vi "index.vi"() -> (1 "XY graph visual":cluster{dbl[], dbl[]}(graph))   [LabVIEW 2026]
uses:
  <userlib>/Status.ctl
  <vilib>/Instr/_visa.llb/VISA Flush IO Buffer Mask.ctl
  <vilib>/Instr/_visa.llb/VISA Configure Serial Port (Instr).vi
  <vilib>/Analysis/3filter.llb/Butterworth Filter (DBL).vi
  <vilib>/measure/maspectr.llb/FFT Spectrum (Mag-Phase) for N Chan.vi
  <vilib>/measure/NI_MAPro.lvlib
  <vilib>/Analysis/NI_AALBase.lvlib
panel:
  in  "Okno osy X":dbl(knob) scale=5.0..30.0 scale format="%#_4g"
  in  "DO 2":bool
  in  "DO 1":bool
  in  "Cluster 2":T1={"Zařízení"="", "Cesta k uloženému souboru"=path "", "Vzorkovací frekvence"=enum."1000", "Record Button"=FALSE, "Stop Button"=FALSE, "A1 signál"=enum."EMG", "A2 signál"=enum."EMG", "A3 signál"=enum."EMG", "A4 signál"=enum."EMG", "A5 signál"=enum."EMG", "A6 signál"=enum."EMG", "Pin s připojeným signálem"=enum."A1"}
  out "read buffer":string
  out "CRC Error":bool
  out "Spectrum":cluster{"f0":dbl, "df":dbl, "magnitude":dbl[]}[](graph)
  in  "EditCluster":T2={"Horní mezní frekvence"=0.45000000000000007, "Dolní mezní frekvence"=0.0, "filter type"=enum."Lowpass", "applyFilter"=FALSE, "removeFilter"=FALSE, "undoFIlter"=FALSE} {"Horní mezní frekvence" format="%0.2f"}
  out "Waveform Graph Edit":waveform(dbl)[](graph)
  out "Zobrazeni typu signalu":cluster{string, string}
  in  "Exit Button":bool
  in  "MereniAZpracovaniSwitch":bool
  in  "DO 4":bool
  in  "DO 3":bool
  out "tdms file":refnum<k34>
  out "Ylabel and Plot name":cluster{string, string}
  out "Sample Rate Numeric":i32
  out "Consumer":i32
  out "producer":i32
  in  "error in (no error)":errorcluster
  out "Sync Stop":bool=TRUE
  # "Aplikace pro měření a zpracování dat na platformě PLUX BITalino"
  # "Hz"
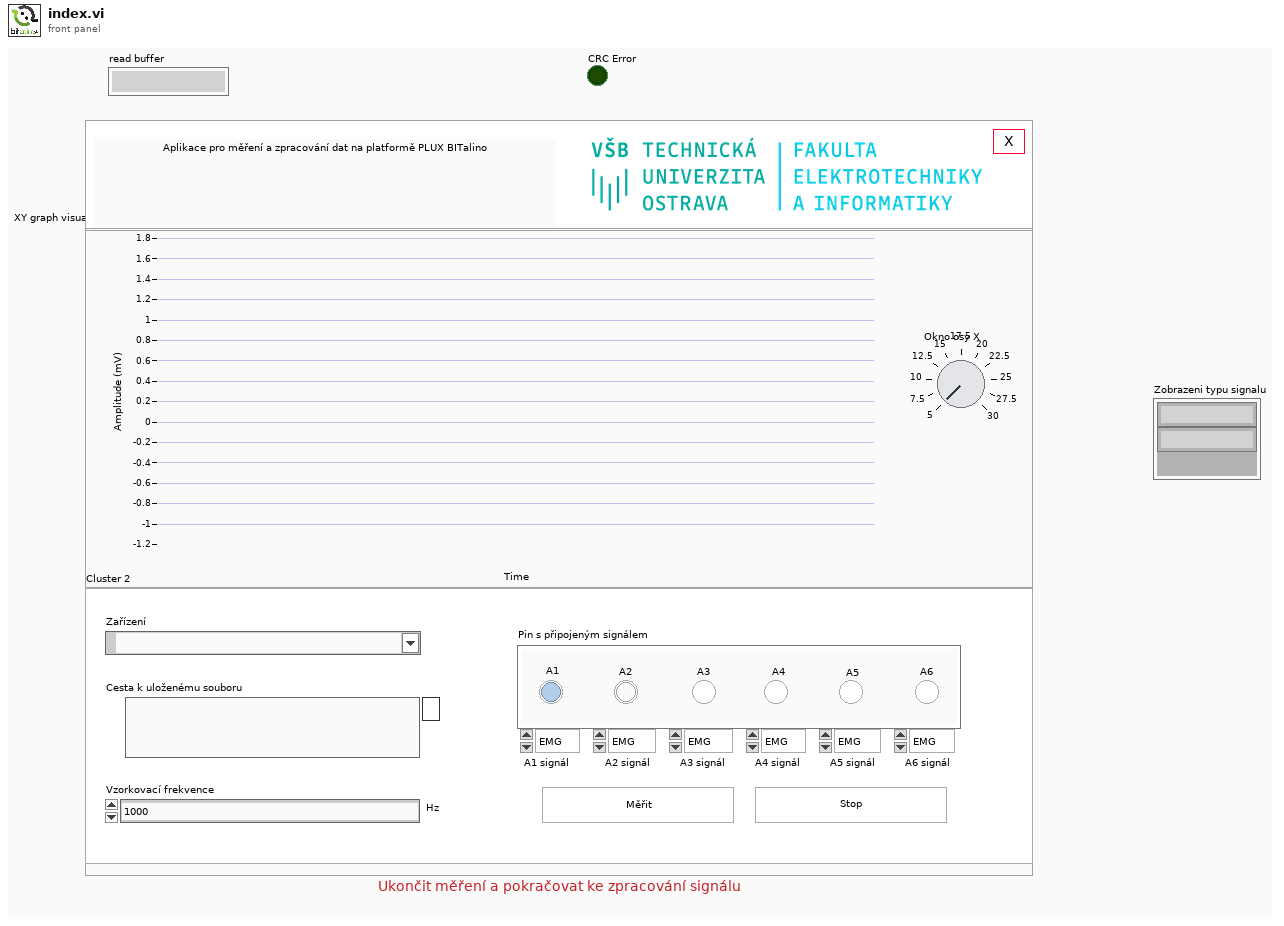
[diagram p1: front panel]
types:
  T1 = cluster{"Zařízení":refnum<visa-resource-name>, "Cesta k uloženému souboru":path, "Vzorkovací frekvence":enum16{"1", "10", "100", "1000"}, "Record Button":bool, "Stop Button":bool, "A1 signál":enum16{"EMG", "ECG", "EEG", "EDA", "ACC"}, "A2 signál":enum16{"EMG", "ECG", "EEG", "EDA", "ACC"}, "A3 signál":enum16{"EMG", "ECG", "EEG", "EDA", "ACC"}, "A4 signál":enum16{"EMG", "ECG", "EEG", "EDA", "ACC"}, "A5 signál":enum16{"EMG", "ECG", "EEG", "EDA", "ACC"}, "A6 signál":enum16{"EMG", "ECG", "EEG", "EDA", "ACC"}, "Pin s připojeným signálem":enum32{"A1", "A2", "A3", "A4", "A5", "A6"}}
  T2 = cluster{"Horní mezní frekvence":dbl, "Dolní mezní frekvence":dbl, "filter type":enum32{"Lowpass", "Highpass", "Bandpass", "Bandstop"}, "applyFilter":bool, "removeFilter":bool, "undoFIlter":bool}
  T3 = enum8{"Enabled", "Disabled", "Disabled and Grayed Out"}
  T4 = enum16{"open", "open or create", "create or replace", "create", "open (read-only)"}
  T5 = typedef "Status.ctl" = enum16{"Initialize", "Edit", "Standby", "Recording", "Exit"}
  T6 = typedef "VISA Flush IO Buffer Mask.ctl" = u16
  T7 = enum32{"Lowpass", "Highpass", "Bandpass", "Bandstop"}
  T8 = cluster{"A1 signál":enum16{"EMG", "ECG", "EEG", "EDA", "ACC"}, "A2 signál":enum16{"EMG", "ECG", "EEG", "EDA", "ACC"}, "A3 signál":enum16{"EMG", "ECG", "EEG", "EDA", "ACC"}, "A4 signál":enum16{"EMG", "ECG", "EEG", "EDA", "ACC"}, "A5 signál":enum16{"EMG", "ECG", "EEG", "EDA", "ACC"}, "A6 signál":enum16{"EMG", "ECG", "EEG", "EDA", "ACC"}}
  T9 = cluster{"Result":dbl, "Result":dbl, "Result":dbl, "Result":dbl, "Result":dbl, "Result":dbl}
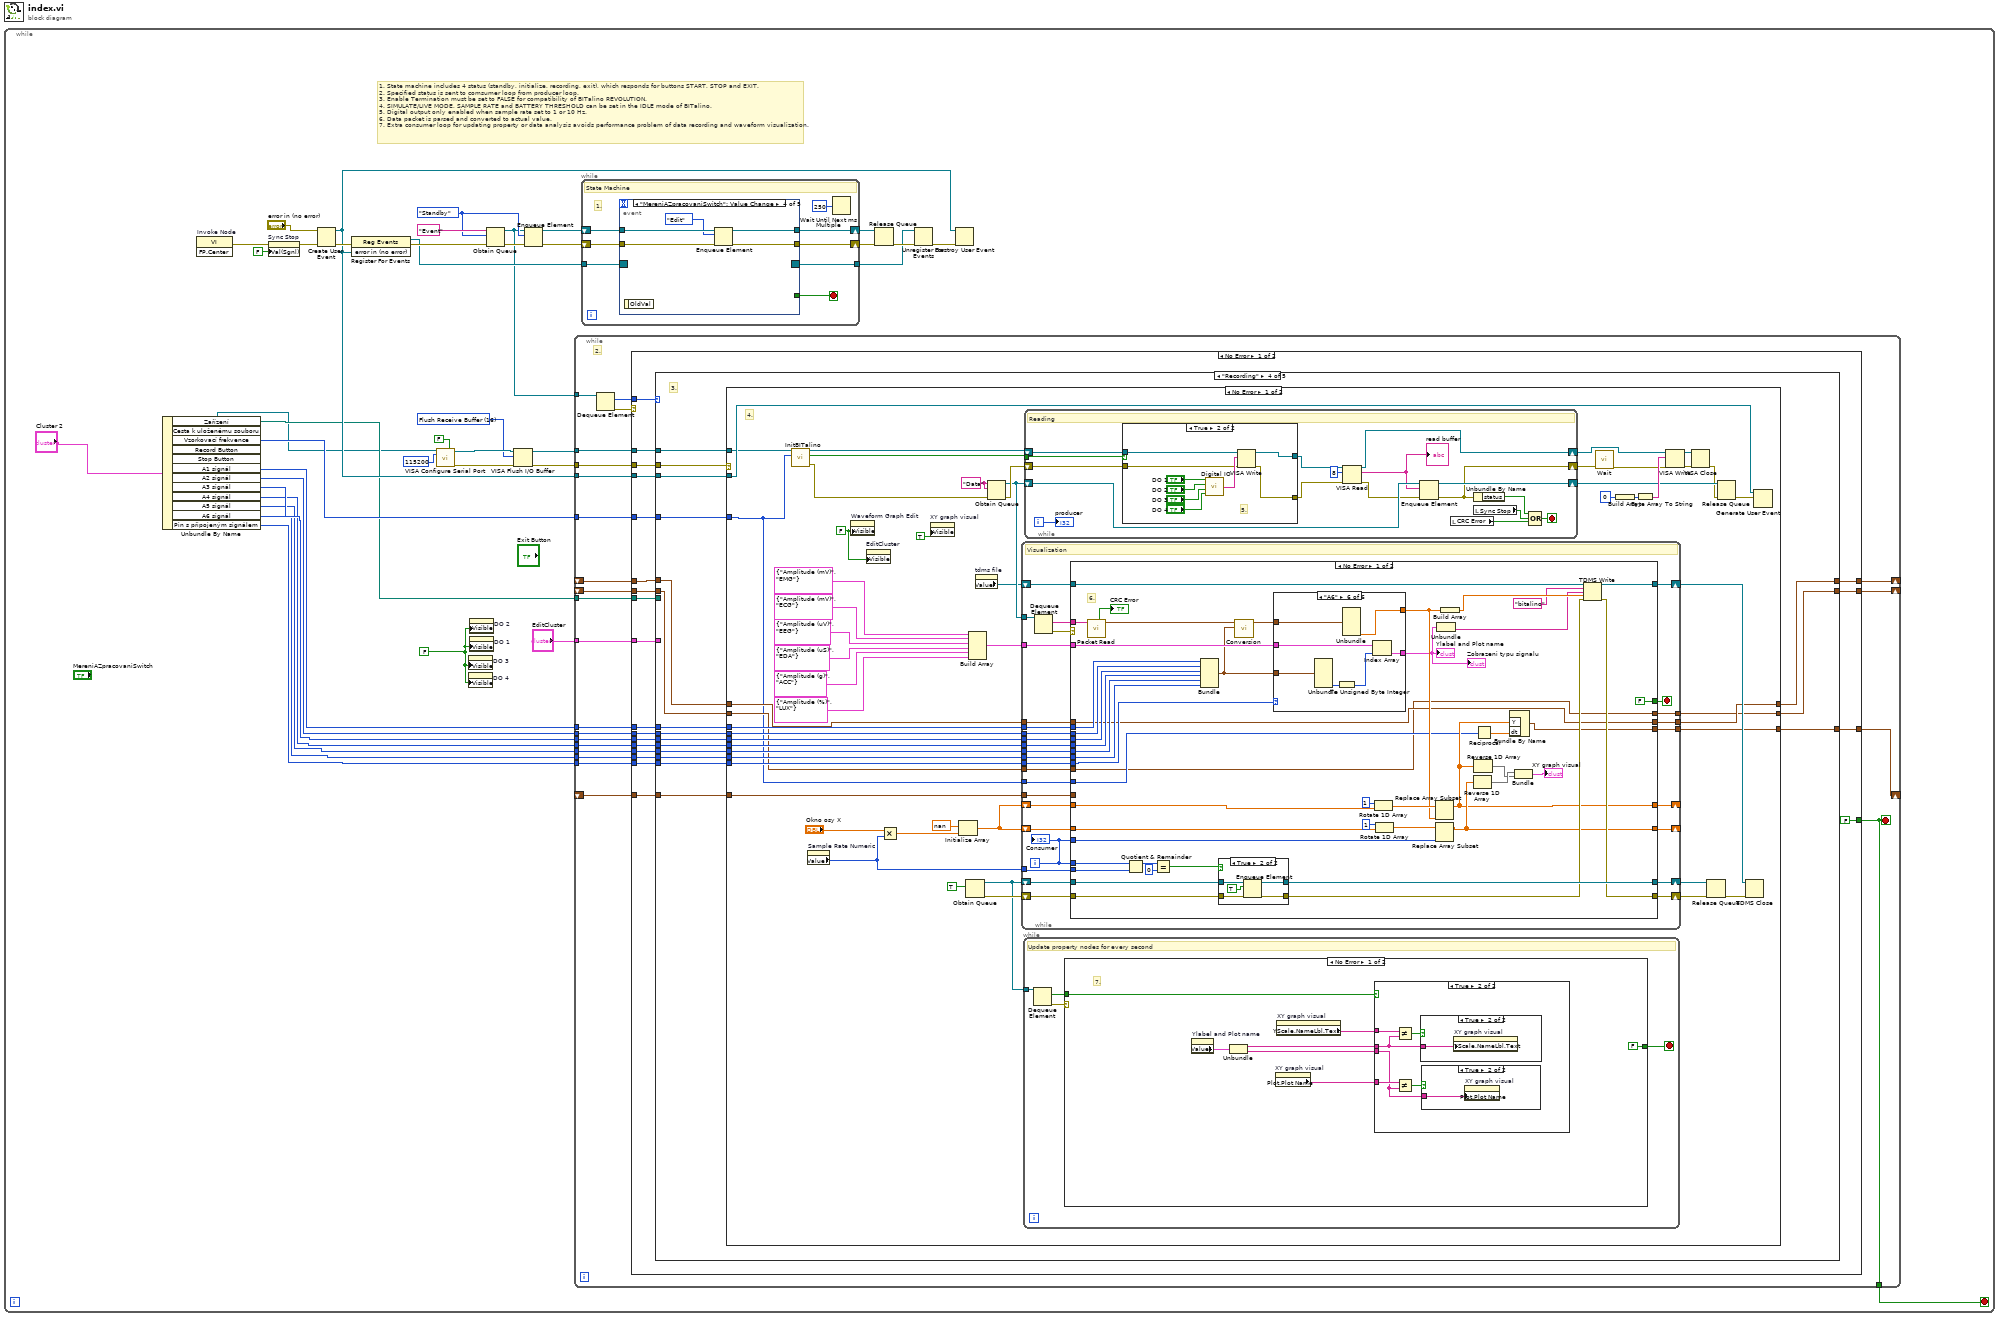
[diagram p0: block diagram]
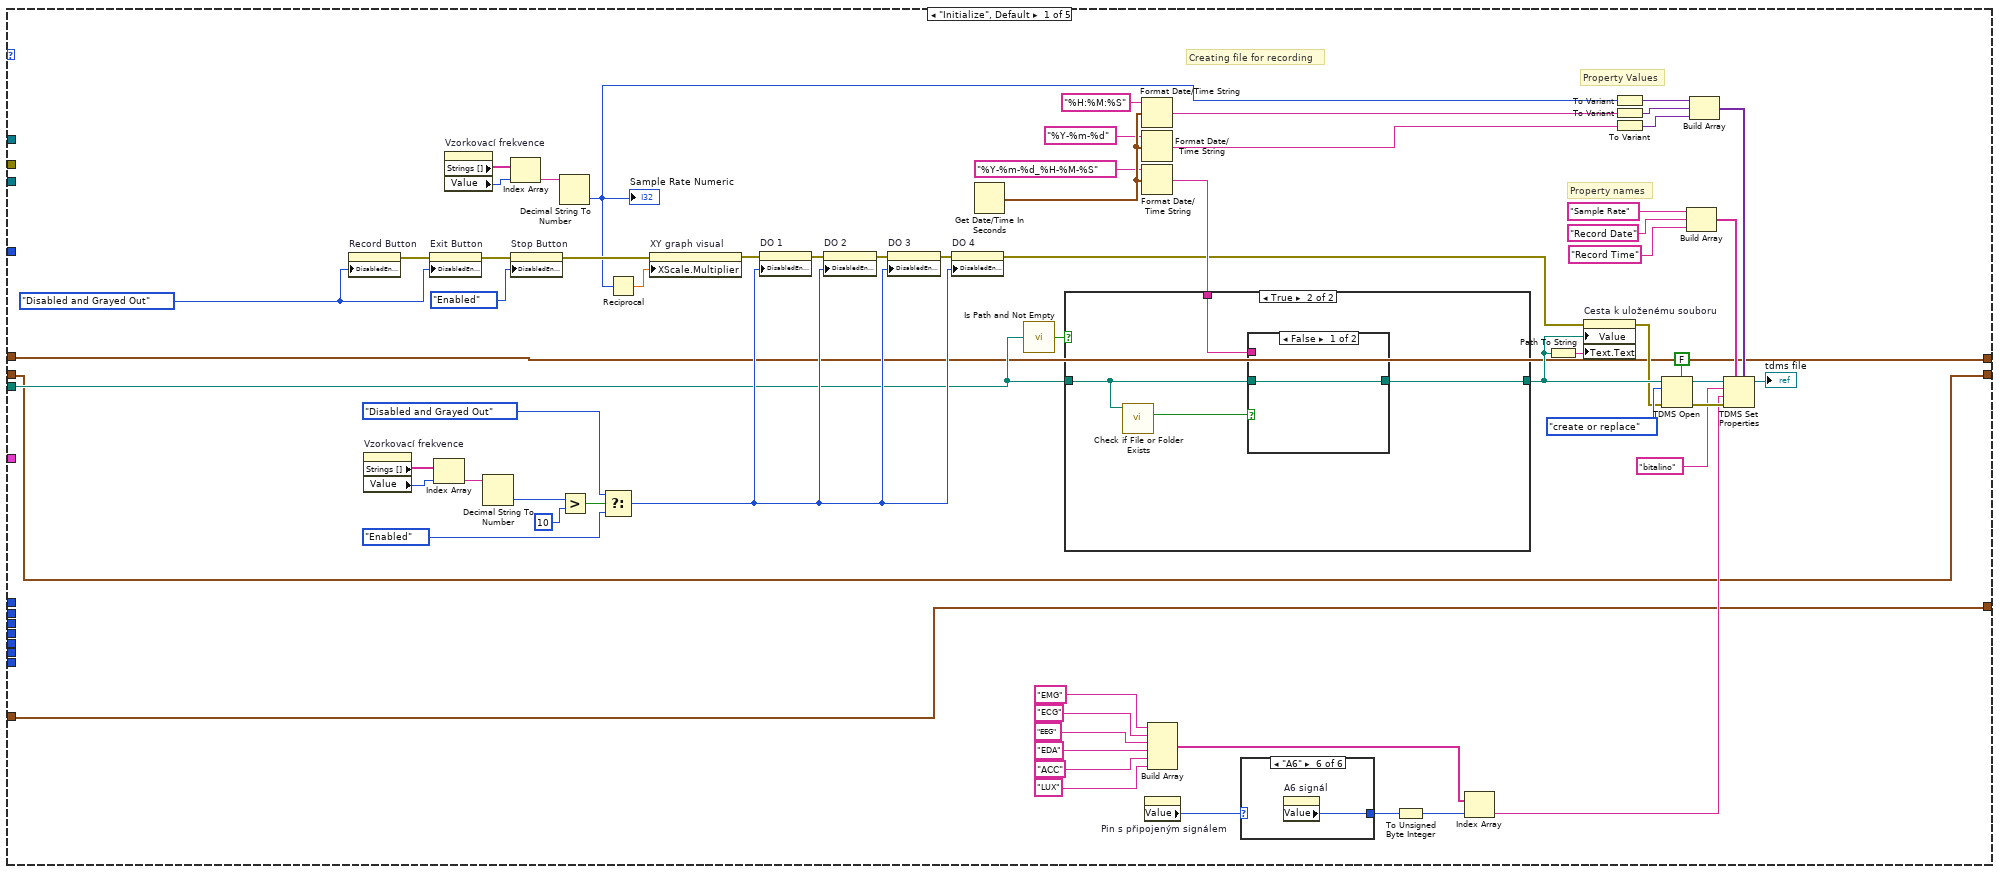
[diagram p2: hidden frame]
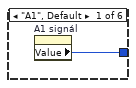
[diagram p3: hidden frame]
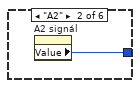
[diagram p4: hidden frame]
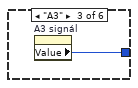
[diagram p5: hidden frame]
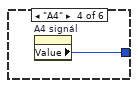
[diagram p6: hidden frame]
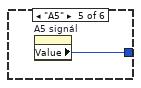
[diagram p7: hidden frame]
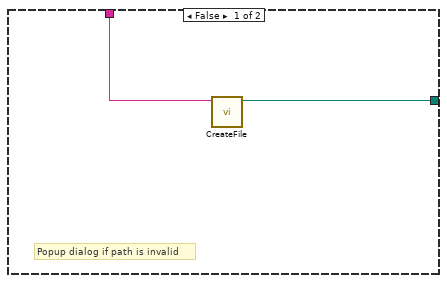
[diagram p8: hidden frame]
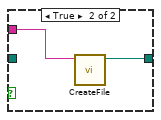
[diagram p9: hidden frame]
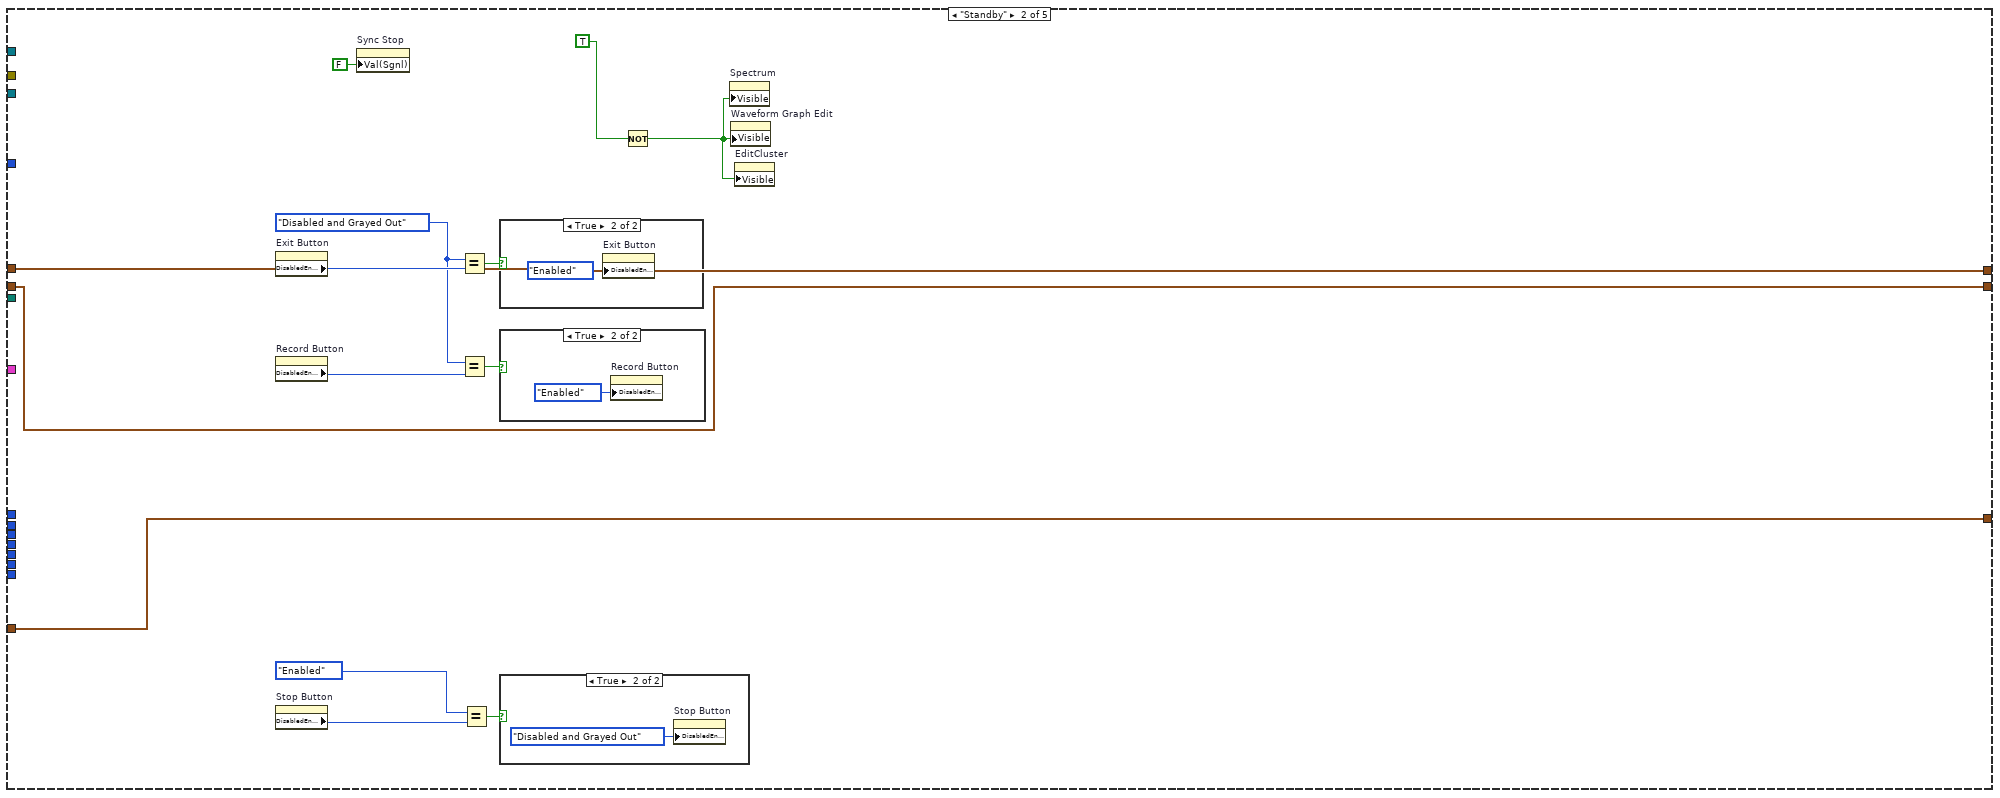
[diagram p10: hidden frame]
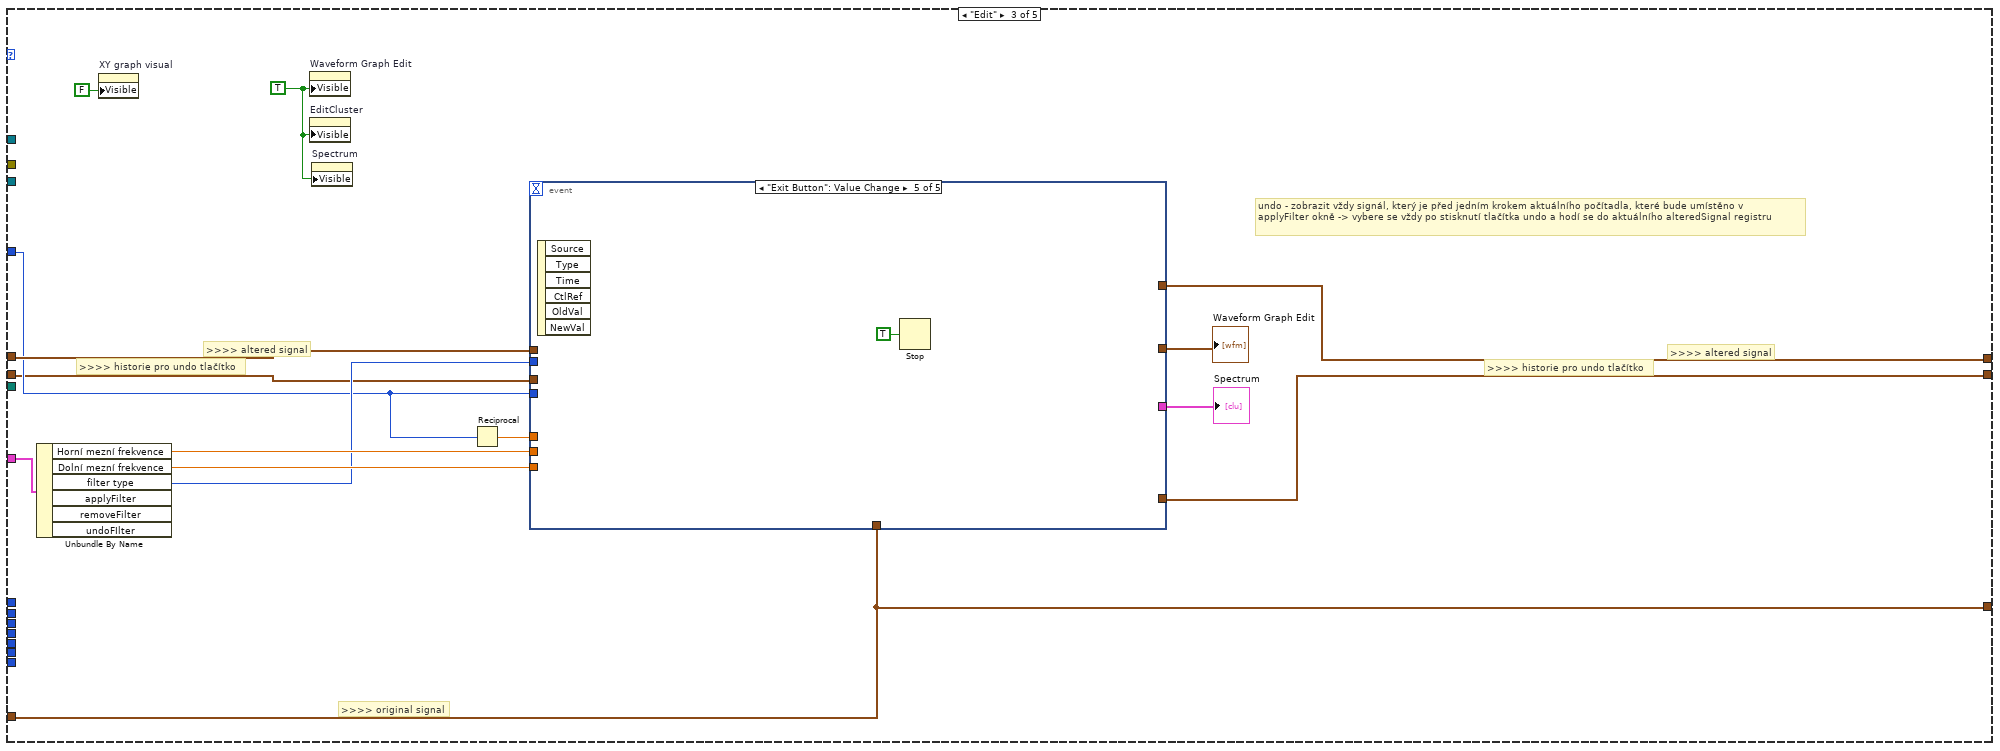
[diagram p14: hidden frame]
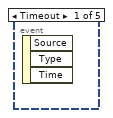
[diagram p15: hidden frame]
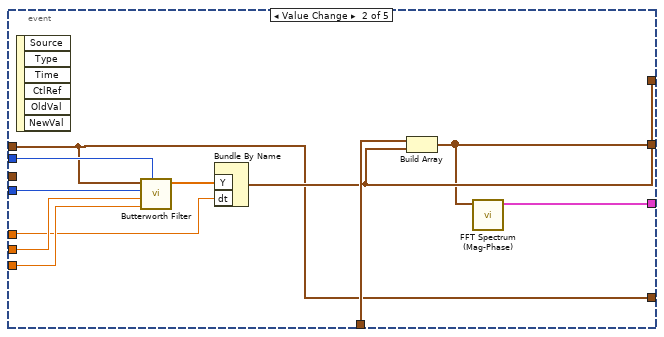
[diagram p16: hidden frame]
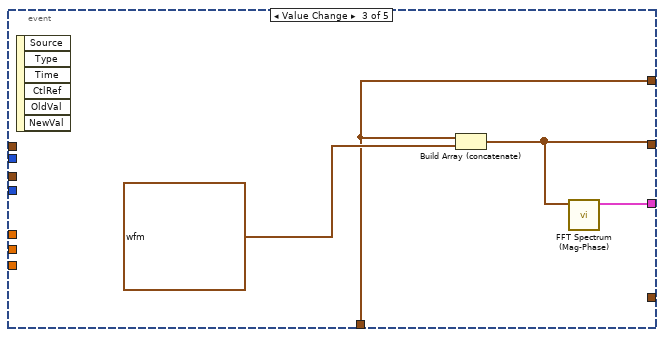
[diagram p17: hidden frame]
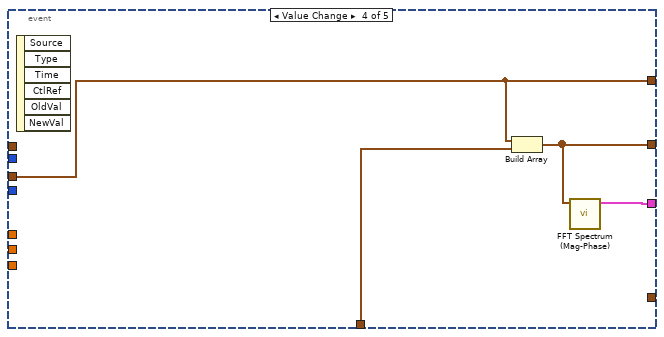
[diagram p18: hidden frame]
diagram:
  n1 = while {
    stop <- w12 stop-if-true
    w1 = FALSE
    w3 = T6 16 items=["Flush Receive Buffer"=16, "Write Transmit Buffer to Device"=32, "Flush Receive Buffer (No I/O)"=64, "Flush Transmit Buffer"=128] ("Mask")
    w39 = Status."Standby" ("Enum")
    # "1. State machine includes 4 status (standby, initialize, recording, exit), which responds for buttons START, STOP and EXIT.\n2. Specified status is sent to comsumer loop from producer loop.\n3. Enable Termination must be set to FALSE for compatibility of BITalino REVOLUTION.\n4. SIMULATE/LIVE MODE, SAMPLE RATE and BATTERY THRESHOLD can be set in the IDLE mode of BITalino.\n5. Digital output only enabled when sample rate set to 1 or 10 Hz.\n6. Data packet is parsed and converted to actual value.\n7. Extra consumer loop for updating property or data analysis avoids performance problem of data recording and waveform visualization."
    n2 = Unbundle By Name("Cluster 2") -> ("Zařízení"=w10:refnum<visa-resource-name>, "Cesta k uloženému souboru"=w13:path, "Vzorkovací frekvence"=w21:enum16{"1", "10", "100", "1000"}, "A1 signál"=w20:enum16{"EMG", "ECG", "EEG", "EDA", "ACC"}, "A2 signál"=w19:enum16{"EMG", "ECG", "EEG", "EDA", "ACC"}, "A3 signál"=w18:enum16{"EMG", "ECG", "EEG", "EDA", "ACC"}, "A4 signál"=w17:enum16{"EMG", "ECG", "EEG", "EDA", "ACC"}, "A5 signál"=w16:enum16{"EMG", "ECG", "EEG", "EDA", "ACC"}, "A6 signál"=w15:enum16{"EMG", "ECG", "EEG", "EDA", "ACC"}, "Pin s připojeným signálem"=w14:enum32{"A1", "A2", "A3", "A4", "A5", "A6"})  [unwired: 2 out]
    n3 = invoke on="Invoke Node" class="VI" method="FP.Center"() -> (error out=w23:errorcluster)  [unwired: 3 in, 2 out]
    n4 = property on="Sync Stop" class="Bool (strict)"(error in=w23, "Val(Sgnl)"=FALSE ("Value (Signaling)")) -> (error out=w32:errorcluster)  [unwired: 1 in, 1 out]
    n5 = Create User Event(user event datatype="error in (no error)", error in=w32) -> (user event=w24:refnum<user-event>, error out=w31:errorcluster)
    n6 = register-events(error in=w31, w24) -> (reference out=w29:refnum<event-registration>, error out=w30:errorcluster)  [unwired: 1 in]
    n7 = call-poly "VISA Configure Serial Port"("VISA resource name"=w10, "Enable Termination\nChar (T)"=FALSE ("Enable Termination\nChar (T)"), "baud rate (9600)"=u32 115200) -> ("VISA resource name out"=w7:refnum<visa-resource-name>, "error out"=w6:errorcluster)  [unwired: 11 in]
    n8 = property on="DO 3" class="Bool (strict)"("Visible"=w1) -> ()  [unwired: 2 in, 2 out]
    n9 = property on="DO 4" class="Bool (strict)"("Visible"=w1) -> ()  [unwired: 2 in, 2 out]
    n10 = property on="DO 2" class="Bool (strict)"("Visible"=w1) -> ()  [unwired: 2 in, 2 out]
    n11 = property on="DO 1" class="Bool (strict)"("Visible"=w1) -> ()  [unwired: 2 in, 2 out]
    n12 = Obtain Queue(name (unnamed)="Event", element data type=w39, error in (no error)=w30) -> (queue out=w22:refnum<queue>, error out=w35:errorcluster)  [unwired: 2 in, 1 out]
    n13 = VISA Flush I/O Buffer(VISA resource name=w7, mask (16)=w3, error in (no error)=w6) -> (VISA resource name out=w5:refnum<visa-resource-name>, error out=w4:errorcluster)
    n14 = Enqueue Element(queue=w22, element=w39, error in (no error)=w35) -> (queue out=w33:refnum<queue>, error out=w34:errorcluster)  [unwired: 1 in, 1 out]
    n15 = while {
      tunnel: w22 -> [w63]
      tunnel: w24 -> [w43]
      tunnel: w21 -> [w60]
      tunnel: [w59] -> w12
      tunnel: w20 -> [w58]
      tunnel: w19 -> [w57]
      tunnel: w18 -> [w56]
      tunnel: w17 -> [w55]
      tunnel: w16 -> [w54]
      tunnel: w15 -> [w53]
      tunnel: w14 -> [w52]
      tunnel: w13 -> [w51]
      shift-right: [w50] -> _
      shift-left: _ -> [w49]
      tunnel: "EditCluster" -> [w48]
      shift-right: [w47] -> _
      shift-left: _ -> [w46]
      shift-right: [w45] -> _
      shift-left: _ -> [w44]
      tunnel: w4 -> [w42]
      tunnel: w5 -> [w41]
      stop <- w59 stop-if-true
      # "2."
      n16 = Dequeue Element(queue=w63) -> (element=w62:T5, error out=w61:errorcluster)  [unwired: 2 in, 2 out]
      n17 = case shown="No Error" w61 {
        tunnel: w62 -> [w82 _]
        tunnel: [FALSE TRUE] -> w59
        tunnel: w60 -> [w83 _]
        tunnel: w58 -> [w81 _]
        tunnel: w57 -> [w80 _]
        tunnel: w56 -> [w79 _]
        tunnel: w55 -> [w78 _]
        tunnel: w54 -> [w77 _]
        tunnel: w53 -> [w76 _]
        tunnel: w52 -> [w75 _]
        tunnel: w51 -> [w74 _]
        tunnel: [w73 w485] -> w50
        tunnel: w49 -> [w72 w485]
        tunnel: w48 -> [w71 _]
        tunnel: [w70 w484] -> w47
        tunnel: w46 -> [w69 w484]
        tunnel: [w68 w483] -> w45
        tunnel: w44 -> [w67 w483]
        tunnel: w43 -> [w66 _]
        tunnel: w42 -> [w65 _]
        tunnel: w41 -> [w64 _]
        frame No Error {
          n18 = case shown="\"Recording\"" w82 {
            tunnel: w83 -> [_ _ w187 w232 _]
            tunnel: w81 -> [_ _ _ w231 _]
            tunnel: w80 -> [_ _ _ w230 _]
            tunnel: w79 -> [_ _ _ w229 _]
            tunnel: w78 -> [_ _ _ w228 _]
            tunnel: w77 -> [_ _ _ w227 _]
            tunnel: w76 -> [_ _ _ w226 _]
            tunnel: w75 -> [_ _ _ w225 _]
            tunnel: w74 -> [w88 _ _ _ _]
            tunnel: [w87 w168 w184 w224 w480] -> w73
            tunnel: w72 -> [w87 w168 w184 w223 w480]
            tunnel: w71 -> [_ _ w194 _ _]
            tunnel: [w86 w167 w183 w222 w479] -> w70
            tunnel: w69 -> [w86 w167 w192 w221 w479]
            tunnel: [w85 w165 w182 w220 w478] -> w68
            tunnel: w67 -> [w85 w165 w181 w219 w478]
            tunnel: w66 -> [_ _ _ w218 _]
            tunnel: w65 -> [_ _ _ w217 _]
            tunnel: w64 -> [_ _ _ w216 _]
            frame "Initialize", Default {
              w116 = T3."Disabled and Grayed Out" ("Disabled")
              # "Creating file for recording"
              # "Property Values"
              # "Property names"
              n19 = property on="Record Button" class="Bool"("DisabledEnum"=w116) -> (error out=w148:errorcluster)  [unwired: 2 in, 1 out]
              n20 = property on="Vzorkovací frekvence" class="Enum (strict)"() -> ("Strings []"=w106:string[], "Value"=w105:enum16{"1", "10", "100", "1000"})  [unwired: 2 in, 2 out]
              n21 = property on="Exit Button" class="Bool"(error in=w148, "DisabledEnum"=w116) -> (error out=w146:errorcluster)  [unwired: 1 in, 1 out]
              n22 = Index Array "Index Array"(array=w106, index=w105) -> (element=w104:string)
              n23 = property on="Vzorkovací frekvence" class="Enum (strict)"() -> ("Strings []"=w145:string[], "Value"=w144:enum16{"1", "10", "100", "1000"})  [unwired: 2 in, 2 out]
              n24 = Decimal String To Number(string=w104) -> (number=w103:i32)  [unwired: 2 in, 1 out]
              n25 = Index Array(array=w145, index=w144) -> (element=w143:string)
              n26 = property on="Stop Button" class="Bool"(error in=w146, "DisabledEnum"=T3."Enabled" ("Disabled")) -> (error out=w142:errorcluster)  [unwired: 1 in, 1 out]
              n27 = Decimal String To Number(string=w143) -> (number=w115:i32)  [unwired: 2 in, 1 out]
              "Sample Rate Numeric" <- w115
              n28 = Greater?(x=w103, y=10) -> (0:w111:bool)
              n29 = Select(t=T3."Disabled and Grayed Out" ("Disabled"), s=w111, f=T3."Enabled" ("Disabled")) -> (s? t:f=w114:T3)
              n30 = Reciprocal(x=w115) -> (1/x=w141:dbl)
              n31 = property on="XY graph visual" class="XYGraph (strict)"(error in=w142, "XScale.Multiplier"=w141) -> (error out=w102:errorcluster)  [unwired: 1 in, 1 out]
              n32 = property on="DO 1" class="Bool (strict)"(error in=w102, "DisabledEnum"=w114) -> (error out=w109:errorcluster)  [unwired: 1 in, 1 out]
              n33 = property on="DO 2" class="Bool (strict)"(error in=w109, "DisabledEnum"=w114) -> (error out=w108:errorcluster)  [unwired: 1 in, 1 out]
              n34 = property on="DO 3" class="Bool (strict)"(error in=w108, "DisabledEnum"=w114) -> (error out=w107:errorcluster)  [unwired: 1 in, 1 out]
              n35 = property on="DO 4" class="Bool (strict)"(error in=w107, "DisabledEnum"=w114) -> (error out=w101:errorcluster)  [unwired: 1 in, 1 out]
              n36 = Get Date/Time In Seconds() -> (seconds since 1Jan1904=w131:timestamp)
              n37 = call <vilib>:"Is Path and Not Empty.vi"("path"=w88) -> ("Is Path and Not Empty?"=w123:bool)  [unwired: 4 in]
              n38 = Format Date/Time String(time format string (%c)="%H:%M:%S", seconds (now)=w131) -> (date/time string=w136:string)  [unwired: 1 in]
              n39 = Format Date/Time String(time format string (%c)="%Y-%m-%d", seconds (now)=w131) -> (date/time string=w137:string)  [unwired: 1 in]
              n40 = Format Date/Time String(time format string (%c)="%Y-%m-%d_%H-%M-%S", seconds (now)=w131) -> (date/time string=w127:string)  [unwired: 1 in]
              n41 = case shown="True" w123 {
                tunnel: [w155 w158] -> w120
                tunnel: w88 -> [_ w157]
                tunnel: w127 -> [w156 w159]
                frame False {
                  # "Popup dialog if path is invalid"
                  n42 = call "CreateFile.vi"("date/time string"=w156) -> ("appended path"=w155:path)  [unwired: 10 in]
                }
                frame True {
                  n43 = call <vilib>:"Check if File or Folder Exists.vi"("path"=w157) -> ("file or folder exists?"=w160:bool)  [unwired: 8 in, 2 out]
                  n44 = case shown="False" w160 {
                    tunnel: w159 -> [_ w163]
                    tunnel: [w161 w162] -> w158
                    tunnel: w157 -> [w161 _]
                    frame False {
                    }
                    frame True {
                      n45 = call "CreateFile.vi"("date/time string"=w163) -> ("appended path"=w162:path)  [unwired: 10 in]
                    }
                  }
                }
              }
              n46 = property on="Pin s připojeným signálem" class="RadioBtnsControl (strict)"() -> ("Value"=w99:enum32{"A1", "A2", "A3", "A4", "A5", "A6"})  [unwired: 2 in, 2 out]
              n47 = Build Array("EMG", "ECG", "EEG", "EDA", "ACC", "LUX") -> (w90:string[])
              n48 = case shown="\"A6\"" w99 {
                tunnel: [w149 w150 w151 w152 w153 w154] -> w92
                frame "A1", Default {
                  n49 = property on="A1 signál" class="Enum (strict)"() -> ("Value"=w149:enum16{"EMG", "ECG", "EEG", "EDA", "ACC"})  [unwired: 2 in, 2 out]
                }
                frame "A2" {
                  n50 = property on="A2 signál" class="Enum (strict)"() -> ("Value"=w150:enum16{"EMG", "ECG", "EEG", "EDA", "ACC"})  [unwired: 2 in, 2 out]
                }
                frame "A3" {
                  n51 = property on="A3 signál" class="Enum (strict)"() -> ("Value"=w151:enum16{"EMG", "ECG", "EEG", "EDA", "ACC"})  [unwired: 2 in, 2 out]
                }
                frame "A4" {
                  n52 = property on="A4 signál" class="Enum (strict)"() -> ("Value"=w152:enum16{"EMG", "ECG", "EEG", "EDA", "ACC"})  [unwired: 2 in, 2 out]
                }
                frame "A5" {
                  n53 = property on="A5 signál" class="Enum (strict)"() -> ("Value"=w153:enum16{"EMG", "ECG", "EEG", "EDA", "ACC"})  [unwired: 2 in, 2 out]
                }
                frame "A6" {
                  n54 = property on="A6 signál" class="Enum (strict)"() -> ("Value"=w154:enum16{"EMG", "ECG", "EEG", "EDA", "ACC"})  [unwired: 2 in, 2 out]
                }
              }
              n55 = To Unsigned Byte Integer(number=w92) -> (unsigned 8bit integer=w91:u8)
              n56 = Index Array(array=w90, index=w91) -> (element=w89:string)
              n57 = Path To String(path=w120) -> (string=w121:string)
              n58 = property on="Cesta k uloženému souboru" class="Path"(error in=w101, "Value"=w120, "Text.Text"=w121) -> (error out=w119:errorcluster)  [unwired: 1 in, 1 out]
              n59 = To Variant(anything=w115) -> (Variant=w135:variant)
              n60 = To Variant(anything=w136) -> (Variant=w138:variant)
              n61 = To Variant(anything=w137) -> (Variant=w139:variant)
              n62 = TDMS Open(5:FALSE ("create index file? (T)"), 8:w119, 10:T4."create or replace" ("operation (0:open)"), 11:w120) -> (0:w126:errorcluster, 3:w125:refnum<k34>)  [unwired: 3 in]
              n63 = Build Array("Sample Rate", "Record Date", "Record Time") -> (w134:string[])
              n64 = Build Array(w135, w138, w139) -> (w140:variant[])
              n65 = TDMS Set Properties(5:w140, 7:w134, 8:w126, 9:w89, 10:"bitalino", 11:w125) -> (3:→"tdms file":refnum<k34>)  [unwired: 3 out]
            }
            frame "Standby" {
              w169 = T3."Disabled and Grayed Out" ("Disabled")
              n66 = property on="Exit Button" class="Bool"() -> ("DisabledEnum"=w176:T3)  [unwired: 2 in, 2 out]
              n67 = property on="Record Button" class="Bool"() -> ("DisabledEnum"=w174:T3)  [unwired: 2 in, 2 out]
              n68 = property on="Stop Button" class="Bool"() -> ("DisabledEnum"=w171:T3)  [unwired: 2 in, 2 out]
              n69 = property on="Sync Stop" class="Bool (strict)"("Val(Sgnl)"=FALSE ("Value (Signaling)")) -> ()  [unwired: 2 in, 2 out]
              n70 = Equal?(x=w169, y=w176) -> (x = y?=w175:bool)
              n71 = Equal?(x=w169, y=w174) -> (x = y?=w173:bool)
              n72 = Equal?(x=T3."Enabled" ("Disabled"), y=w171) -> (x = y?=w170:bool)
              n73 = case shown="True" w175 {
                frame False {
                }
                frame True {
                  n74 = property on="Exit Button" class="Bool"("DisabledEnum"=T3."Enabled" ("Disabled")) -> ()  [unwired: 2 in, 2 out]
                }
              }
              n75 = case shown="True" w173 {
                frame False {
                }
                frame True {
                  n76 = property on="Record Button" class="Bool"("DisabledEnum"=T3."Enabled" ("Disabled")) -> ()  [unwired: 2 in, 2 out]
                }
              }
              n77 = case shown="True" w170 {
                frame False {
                }
                frame True {
                  n78 = property on="Stop Button" class="Bool"("DisabledEnum"=T3."Disabled and Grayed Out" ("Disabled")) -> ()  [unwired: 2 in, 2 out]
                }
              }
              n79 = Not(x=TRUE ("Visible")) -> (.not. x?=w166:bool)
              n80 = property on="Spectrum" class="WFGraph (strict)"("Visible"=w166) -> ()  [unwired: 2 in, 2 out]
              n81 = property on="Waveform Graph Edit" class="WFGraph (strict)"("Visible"=w166) -> ()  [unwired: 2 in, 2 out]
              n82 = property on="EditCluster" class="Clust"("Visible"=w166) -> ()  [unwired: 2 in, 2 out]
            }
            frame "Edit" {
              w193 = TRUE ("Visible")
              # ">>>> altered signal"
              # ">>>> historie pro undo tlačítko"
              # ">>>> historie pro undo tlačítko"
              # "undo - zobrazit vždy signál, který je před jedním krokem aktuálního počítadla, které bude umístěno v \napplyFilter okně -> vybere se vždy po stisknutí tlačítka undo a hodí se do aktuálního alteredSignal registru"
              # ">>>> altered signal"
              # ">>>> original signal"
              n83 = Unbundle By Name(w194) -> ("Horní mezní frekvence"=w190:dbl, "Dolní mezní frekvence"=w189:dbl, "filter type"=w188:T7)  [unwired: 3 out]
              n84 = property on="XY graph visual" class="XYGraph (strict)"("Visible"=FALSE) -> ()  [unwired: 2 in, 2 out]
              n85 = property on="Waveform Graph Edit" class="WFGraph (strict)"("Visible"=w193) -> ()  [unwired: 2 in, 2 out]
              n86 = property on="EditCluster" class="Clust"("Visible"=w193) -> ()  [unwired: 2 in, 2 out]
              n87 = property on="Spectrum" class="WFGraph (strict)"("Visible"=w193) -> ()  [unwired: 2 in, 2 out]
              n88 = Reciprocal(x=w187) -> (1/x=w191:dbl)
              n89 = event shown="[4] \"Exit Button\": Value Change" {
                selector: _ -> [_ _ _ _ _]
                dyn-events: _ -> [_ _ _ _ _]
                timeout: _ -> [_ _ _ _ _]
                tunnel: w184 -> [_ w205 w207 w213 _]
                tunnel: [_ w204 w207 w214 _] -> w183
                tunnel: w192 -> [_ w196 _ _ _]
                tunnel: w191 -> [_ w200 _ _ _]
                tunnel: w190 -> [_ w203 _ _ _]
                tunnel: w189 -> [_ w202 _ _ _]
                tunnel: w188 -> [_ w201 _ _ _]
                tunnel: w187 -> [_ w199 _ _ _]
                tunnel: [_ w198 w208 w211 _] -> w186
                tunnel: [_ w197 w209 w212 _] -> w185
                tunnel: [_ w196 _ _ _] -> w182
                tunnel: w181 -> [_ _ _ w214 _]
                event Timeout {
                  n90 = event-data() -> ()  [unwired: 1 in, 3 out]
                }
                event "EditCluster.applyFilter": Value Change {
                  n91 = event-data() -> ()  [unwired: 1 in, 6 out]
                  n92 = call-poly <vilib>:"Butterworth Filter.vi"("filter type"=w201, "low cutoff freq: fl"=w202, "high cutoff freq: fh"=w203, "sampling freq: fs"=w199, "X"=w196) -> ("Filtered X"=w206:dbl[])  [unwired: 3 in, 1 out]
                  n93 = Bundle By Name("Y"=w206, "dt"=w200) -> (w204:waveform(dbl))  [unwired: 1 in]
                  n94 = Build Array(w205, w204) -> (w198:waveform(dbl)[])
                  n95 = call-poly <vilib>:"FFT Spectrum (Mag-Phase).vi"("time signals"=w198) -> ("magnitudes"=w197:cluster{"f0":dbl, "df":dbl, "magnitude":dbl[]}[])  [unwired: 6 in, 4 out]
                }
                event "EditCluster.removeFilter": Value Change {
                  n96 = event-data() -> ()  [unwired: 1 in, 6 out]
                  n97 = Build Array (concatenate)(w207, waveform(dbl)[] [{"t0"=timestamp(-3600 s since 1904-01-01), "dt"=10000.0, "Y"=[0.0]}] ("array")) -> (w208:waveform(dbl)[])
                  n98 = call-poly <vilib>:"FFT Spectrum (Mag-Phase).vi"("time signals"=w208) -> ("magnitudes"=w209:cluster{"f0":dbl, "df":dbl, "magnitude":dbl[]}[])  [unwired: 6 in, 4 out]
                }
                event "EditCluster.undoFIlter": Value Change {
                  n99 = event-data() -> ()  [unwired: 1 in, 6 out]
                  n100 = Build Array(w214, w213) -> (w211:waveform(dbl)[])
                  n101 = call-poly <vilib>:"FFT Spectrum (Mag-Phase).vi"("time signals"=w211) -> ("magnitudes"=w212:cluster{"f0":dbl, "df":dbl, "magnitude":dbl[]}[])  [unwired: 6 in, 4 out]
                }
                event "Exit Button": Value Change {
                  n102 = event-data() -> ()  [unwired: 1 in, 6 out]
                  n103 = Stop(stop? (T)=TRUE) -> ()
                }
              }
              "Waveform Graph Edit" <- w186
              "Spectrum" <- w185
            }
            frame "Recording" {
              # "3."
              n104 = case shown="No Error" w217 {
                selector: w217 -> [_ w476]
                tunnel: w218 -> [w274 w477]
                tunnel: w232 -> [w235 _]
                tunnel: w231 -> [w253 _]
                tunnel: w230 -> [w252 _]
                tunnel: w229 -> [w251 _]
                tunnel: w228 -> [w250 _]
                tunnel: w227 -> [w249 _]
                tunnel: w226 -> [w248 _]
                tunnel: w225 -> [w247 _]
                tunnel: [w246 w475] -> w224
                tunnel: w223 -> [w244 w475]
                tunnel: [w243 w474] -> w222
                tunnel: w221 -> [w242 w474]
                tunnel: [w240 w473] -> w220
                tunnel: w219 -> [w239 w473]
                tunnel: w216 -> [w238 _]
                frame No Error {
                  w241 = FALSE ("Visible")
                  w282 = "Data"
                  # "4."
                  n105 = call "InitBITalino.vi"("Sample Rate"=w235, "BITalino"=w238) -> ("error out"=w234:errorcluster, "Digital Output"=w236:bool, "VISA out"=w237:refnum<visa-resource-name>)  [unwired: 7 in]
                  n106 = property on="Sample Rate Numeric" class="DigNum (strict)"() -> ("Value"=w267:i32)  [unwired: 2 in, 2 out]
                  n107 = property on="Waveform Graph Edit" class="WFGraph (strict)"("Visible"=w241) -> ()  [unwired: 2 in, 2 out]
                  n108 = property on="EditCluster" class="Clust"("Visible"=w241) -> ()  [unwired: 2 in, 2 out]
                  n109 = Multiply(x="Okno osy X", y=w267) -> (x*y=w265:dbl)
                  n110 = property on="XY graph visual" class="XYGraph (strict)"("Visible"=TRUE) -> ()  [unwired: 2 in, 2 out]
                  n111 = Initialize Array(nan ("element"), w265) -> (w264:dbl[])
                  n112 = Obtain Queue(element data type=TRUE) -> (queue out=w270:refnum<queue>, error out=w272:errorcluster)  [unwired: 4 in, 1 out]
                  n113 = Build Array(cluster{string, string} {"Amplitude (mV)", "EMG"}, cluster{string, string} {"Amplitude (mV)", "ECG"}, cluster{string, string} {"Amplitude (uV)", "EEG"}, cluster{string, string} {"Amplitude (uS)", "EDA"}, cluster{string, string} {"Amplitude (g)", "ACC"}, cluster{string, string} {"Amplitude (%)", "LUX"}) -> (w257:cluster{string, string}[])
                  n114 = property on="tdms file" class="Ref (strict)"() -> ("Value"=w256:refnum<k34>)  [unwired: 2 in, 2 out]
                  n115 = Obtain Queue(name (unnamed)=w282, element data type=w282, error in (no error)=w234) -> (queue out=w283:refnum<queue>, error out=w284:errorcluster)  [unwired: 2 in, 1 out]
                  n116 = while {
                    tunnel: w283 -> [w338]
                    shift-right: [w333] -> _
                    shift-left: w264 -> [w334]
                    tunnel: w267 -> [w332]
                    shift-right: [w329] -> w269
                    shift-left: w270 -> [w331]
                    shift-right: [w328] -> w268
                    shift-left: w272 -> [w330]
                    shift-right: [w325] -> _
                    shift-left: w264 -> [w327]
                    tunnel: w257 -> [w324]
                    shift-right: [w322] -> w254
                    shift-left: w256 -> [w323]
                    tunnel: w253 -> [w321]
                    tunnel: w252 -> [w320]
                    tunnel: w251 -> [w319]
                    tunnel: w250 -> [w318]
                    tunnel: w249 -> [w317]
                    tunnel: w248 -> [w316]
                    tunnel: w247 -> [w315]
                    tunnel: w235 -> [w314]
                    tunnel: [w313] -> w246
                    tunnel: w244 -> [w312]
                    tunnel: [w311] -> w243
                    tunnel: w242 -> [w310]
                    tunnel: [w309] -> w240
                    tunnel: w239 -> [w308]
                    i -> [w326]
                    stop <- w336 stop-if-true
                    # "Visualization"
                    n117 = Dequeue Element(queue=w338) -> (element=w335:string, error out=w337:errorcluster)  [unwired: 2 in, 2 out]
                    n118 = case shown="No Error" w337 {
                      tunnel: [FALSE TRUE] -> w336
                      tunnel: w335 -> [w361 _]
                      tunnel: w334 -> [w374 w443]
                      tunnel: [w347 w443] -> w333
                      tunnel: w332 -> [w375 _]
                      tunnel: w326 -> [w380 _]
                      tunnel: w331 -> [w383 w442]
                      tunnel: w330 -> [w382 w441]
                      tunnel: [w381 w442] -> w329
                      tunnel: [w362 w441] -> w328
                      tunnel: w327 -> [w371 w440]
                      tunnel: w326 -> [w370 _]
                      tunnel: [w350 w440] -> w325
                      tunnel: w324 -> [w369 _]
                      tunnel: w323 -> [w367 w439]
                      tunnel: [w366 w439] -> w322
                      tunnel: w321 -> [w357 _]
                      tunnel: w320 -> [w356 _]
                      tunnel: w319 -> [w355 _]
                      tunnel: w318 -> [w354 _]
                      tunnel: w317 -> [w353 _]
                      tunnel: w316 -> [w352 _]
                      tunnel: w315 -> [w351 _]
                      tunnel: w314 -> [w345 _]
                      tunnel: [w344 w438] -> w313
                      tunnel: w312 -> [_ w438]
                      tunnel: [w343 w437] -> w311
                      tunnel: w310 -> [w343 w437]
                      tunnel: [w342 w436] -> w309
                      tunnel: w308 -> [w342 w436]
                      frame No Error {
                        # "6."
                        n119 = call "Packet Read.vi"("Packets"=w361) -> ("Analog Channels"=w360:cluster{u16, u16, u16, u16, u16, u16}, "CRC Error"=→"CRC Error":bool)  [unwired: 7 in, 2 out]
                        n120 = Quotient & Remainder(x=w380, y=w375) -> (x-y*floor(x/y)=w379:i32)  [unwired: 1 out]
                        n121 = Equal?(x=w379, y=0) -> (x = y?=w377:bool)
                        n122 = Bundle "Bundle"("A1 signál"=w357, "A2 signál"=w356, "A3 signál"=w355, "A4 signál"=w354, "A5 signál"=w353, "A6 signál"=w352) -> (w368:T8)  [unwired: 1 in]
                        n123 = case shown="True" w377 {
                          tunnel: w383 -> [w388 w393]
                          tunnel: w382 -> [w387 w392]
                          tunnel: [w388 w391] -> w381
                          tunnel: [w387 w390] -> w365
                          frame False {
                          }
                          frame True {
                            n124 = Enqueue Element(queue=w393, element=TRUE, error in (no error)=w392) -> (queue out=w391:refnum<queue>, error out=w390:errorcluster)  [unwired: 1 in, 1 out]
                          }
                        }
                        n125 = call "Conversion.vi"("Sensor Type"=w368, "Analog Channels"=w360) -> ("Converted Values"=w385:T9)  [unwired: 8 in, 1 out]
                        n126 = case shown="\"A6\"" w351 {
                          tunnel: w385 -> [w400 w407 w414 w421 w428 w435]
                          tunnel: [w399 w406 w413 w420 w427 w434] -> w364
                          tunnel: w369 -> [w395 w402 w409 w417 w423 w431]
                          tunnel: w368 -> [w398 w404 w411 w418 w425 w432]
                          tunnel: [w394 w401 w410 w416 w424 w430] -> w348
                          frame "A1", Default {
                            n127 = Unbundle(w398) -> ("A1 signál"=w396:enum16{"EMG", "ECG", "EEG", "EDA", "ACC"})  [unwired: 5 out]
                            n128 = To Unsigned Byte Integer(number=w396) -> (unsigned 8bit integer=w397:u8)
                            n129 = Unbundle(w400) -> ("Result"=w399:dbl)  [unwired: 5 out]
                            n130 = Index Array(array=w395, index=w397) -> (element=w394:cluster{string, string})
                          }
                          frame "A2" {
                            n131 = Unbundle(w404) -> ("A2 signál"=w403:enum16{"EMG", "ECG", "EEG", "EDA", "ACC"})  [unwired: 5 out]
                            n132 = To Unsigned Byte Integer(number=w403) -> (unsigned 8bit integer=w405:u8)
                            n133 = Unbundle(w407) -> ("Result"=w406:dbl)  [unwired: 5 out]
                            n134 = Index Array(array=w402, index=w405) -> (element=w401:cluster{string, string})
                          }
                          frame "A3" {
                            n135 = Unbundle(w411) -> ("A3 signál"=w408:enum16{"EMG", "ECG", "EEG", "EDA", "ACC"})  [unwired: 5 out]
                            n136 = To Unsigned Byte Integer(number=w408) -> (unsigned 8bit integer=w412:u8)
                            n137 = Unbundle(w414) -> ("Result"=w413:dbl)  [unwired: 5 out]
                            n138 = Index Array(array=w409, index=w412) -> (element=w410:cluster{string, string})
                          }
                          frame "A4" {
                            n139 = Unbundle(w418) -> ("A4 signál"=w415:enum16{"EMG", "ECG", "EEG", "EDA", "ACC"})  [unwired: 5 out]
                            n140 = To Unsigned Byte Integer(number=w415) -> (unsigned 8bit integer=w419:u8)
                            n141 = Unbundle(w421) -> ("Result"=w420:dbl)  [unwired: 5 out]
                            n142 = Index Array(array=w417, index=w419) -> (element=w416:cluster{string, string})
                          }
                          frame "A5" {
                            n143 = Unbundle(w425) -> ("A5 signál"=w422:enum16{"EMG", "ECG", "EEG", "EDA", "ACC"})  [unwired: 5 out]
                            n144 = Unbundle(w428) -> ("Result"=w427:dbl)  [unwired: 5 out]
                            n145 = To Unsigned Byte Integer(number=w422) -> (unsigned 8bit integer=w426:u8)
                            n146 = Index Array(array=w423, index=w426) -> (element=w424:cluster{string, string})
                          }
                          frame "A6" {
                            n147 = Unbundle(w432) -> ("A6 signál"=w429:enum16{"EMG", "ECG", "EEG", "EDA", "ACC"})  [unwired: 5 out]
                            n148 = To Unsigned Byte Integer(number=w429) -> (unsigned 8bit integer=w433:u8)
                            n149 = Unbundle(w435) -> ("Result"=w434:dbl)  [unwired: 5 out]
                            n150 = Index Array(array=w431, index=w433) -> (element=w430:cluster{string, string})
                          }
                        }
                        "Ylabel and Plot name" <- w348
                        "Zobrazeni typu signalu" <- w348
                        n151 = Rotate 1D Array(1:w374, 2:1 ("n")) -> (0:w376:dbl[])
                        n152 = Rotate 1D Array(1:w371, 2:1 ("n")) -> (0:w372:dbl[])
                        n153 = Replace Array Subset(array=w376, new element=w364) -> (w347:dbl[])  [unwired: 1 in]
                        n154 = Replace Array Subset(array=w372, new element=w370) -> (w350:dbl[])  [unwired: 1 in]
                        n155 = Unbundle(w348) -> (w359:string)  [unwired: 1 out]
                        n156 = Build Array(w364) -> (w363:dbl[])
                        n157 = Reverse 1D Array(array=w350) -> (reversed array=w341:dbl[])
                        n158 = Reverse 1D Array(array=w347) -> (reversed array=w340:dbl[])
                        n159 = Reciprocal(x=w345) -> (1/x=w346:dbl)
                        n160 = Bundle By Name("Y"=w347, "dt"=w346) -> (w344:waveform(dbl))  [unwired: 1 in]
                        n161 = Bundle(w341, w340) -> (→"XY graph visual":cluster{dbl[], dbl[]})  [unwired: 1 in]
                        n162 = TDMS Write(0:w367, 5:"bitalino", 7:w359, 9:w363, 11:w365) -> (4:w366:refnum<k34>, 15:w362:errorcluster)  [unwired: 1 in, 2 out]
                      }
                      frame Error {
                      }
                    }
                    "Consumer" <- w326
                  }
                  n163 = while {
                    tunnel: w270 -> [w291]
                    stop <- w288 stop-if-true
                    # "Update property nodes for every second"
                    n164 = Dequeue Element(queue=w291) -> (element=w289:bool, error out=w290:errorcluster)  [unwired: 2 in, 2 out]
                    n165 = case shown="No Error" w290 {
                      tunnel: w289 -> [w295 _]
                      tunnel: [FALSE TRUE] -> w288
                      frame No Error {
                        # "7."
                        n166 = property on="Ylabel and Plot name" class="Clust (strict)"() -> ("Value"=w298:cluster{string, string})  [unwired: 2 in, 2 out]
                        n167 = Unbundle(w298) -> (w297:string, w296:string)
                        n168 = property on="XY graph visual" class="XYGraph (strict)"() -> ("Plot.Plot Name"=w292:string)  [unwired: 2 in, 2 out]
                        n169 = property on="XY graph visual" class="XYGraph (strict)"() -> ("YScale.NameLbl.Text"=w293:string)  [unwired: 2 in, 2 out]
                        n170 = case shown="True" w295 {
                          tunnel: w293 -> [_ w304]
                          tunnel: w292 -> [_ w300]
                          tunnel: w297 -> [_ w301]
                          tunnel: w296 -> [_ w299]
                          frame False {
                          }
                          frame True {
                            n171 = Not Equal?(x=w304, y=w301) -> (x != y?=w302:bool)
                            n172 = Not Equal?(x=w300, y=w299) -> (x != y?=w303:bool)
                            n173 = case shown="True" w302 {
                              tunnel: w301 -> [_ w306]
                              frame False {
                              }
                              frame True {
                                n174 = property on="XY graph visual" class="XYGraph (strict)"("YScale.NameLbl.Text"=w306) -> ()  [unwired: 2 in, 2 out]
                              }
                            }
                            n175 = case shown="True" w303 {
                              tunnel: w299 -> [_ w305]
                              frame False {
                              }
                              frame True {
                                n176 = property on="XY graph visual" class="XYGraph (strict)"("Plot.Plot Name"=w305) -> ()  [unwired: 2 in, 2 out]
                              }
                            }
                          }
                        }
                      }
                      frame Error {
                      }
                    }
                  }
                  n177 = while {
                    shift-right: [w459] -> w278
                    shift-left: w284 -> [w454]
                    shift-right: [w460] -> w281
                    shift-left: w283 -> [w461]
                    shift-right: [w445] -> w280
                    shift-left: w237 -> [w453]
                    tunnel: w236 -> [w452]
                    i -> [w458]
                    stop <- w457 stop-if-true
                    # "Reading"
                    n178 = case shown="True" w452 {
                      tunnel: w454 -> [w463 w469]
                      tunnel: w453 -> [w462 w468]
                      tunnel: [w463 w466] -> w449
                      tunnel: [w462 w467] -> w450
                      frame False {
                      }
                      frame True {
                        # "5."
                        n179 = call "Digital IO.vi"("DO 4"="DO 4", "DO 3"="DO 3", "DO in"="DO 2", "DO 1"="DO 1") -> ("string"=w472:string)
                        n180 = VISA Write(VISA resource name=w468, write buffer=w472, error in (no error)=w469) -> (VISA resource name out=w467:refnum<visa-resource-name>, error out=w466:errorcluster)  [unwired: 1 out]
                      }
                    }
                    n181 = VISA Read(VISA resource name=w450, byte count=u32 8, error in (no error)=w449) -> (VISA resource name out=w445:refnum<visa-resource-name>, read buffer=w447:string, error out=w448:errorcluster)  [unwired: 1 out]
                    "read buffer" <- w447
                    n182 = Enqueue Element(queue=w461, element=w447, error in (no error)=w448) -> (queue out=w460:refnum<queue>, error out=w459:errorcluster)  [unwired: 1 in, 1 out]
                    n183 = local read "CRC Error"() -> (w451:bool)
                    n184 = Unbundle By Name(w459) -> ("status"=w455:bool)
                    n185 = local read "Sync Stop"() -> (w456:bool)
                    n186 = Compound Arithmetic op=OR(w455, w456, w451) -> (w457:bool)
                    "producer" <- w458
                  }
                  n187 = call "Wait.vi"("error in (no error)"=w278) -> ("error out"=w279:errorcluster)  [unwired: 10 in]
                  n188 = Build Array(u8 0) -> (w286:u8[])
                  n189 = Byte Array To String(unsigned byte array=w286) -> (string=w285:string)
                  n190 = VISA Write(VISA resource name=w280, write buffer=w285, error in (no error)=w279) -> (VISA resource name out=w276:refnum<visa-resource-name>, error out=w277:errorcluster)  [unwired: 1 out]
                  n191 = VISA Close(VISA resource name=w276, error in (no error)=w277) -> (error out=w275:errorcluster)
                  n192 = Release Queue(queue=w269, error in (no error)=w268) -> (error out=w255:errorcluster)  [unwired: 1 in, 2 out]
                  n193 = Release Queue(queue=w281, error in (no error)=w275) -> (error out=w273:errorcluster)  [unwired: 1 in, 2 out]
                  n194 = TDMS Close(8:w255, 11:w254) -> ()  [unwired: 2 out]
                  n195 = Generate User Event(user event=w274, event data cluster=w273) -> ()  [unwired: 2 in, 2 out]
                }
                frame Error {
                  n196 = Generate User Event(user event=w477, event data cluster=w476) -> ()  [unwired: 2 in, 2 out]
                }
              }
            }
            frame "Exit" {
              n197 = flat-sequence {
                frame #0 {
                  n198 = property on="Stop Button" class="Bool"("DisabledEnum"=T3."Enabled" ("Disabled")) -> ()  [unwired: 2 in, 2 out]
                }
                frame #1 {
                  n199 = Stop(stop? (T)=TRUE) -> ()
                }
              }
            }
          }
        }
        frame Error {
        }
      }
    }
    n200 = while {
      shift-right: [w491] -> w37
      shift-left: w33 -> [w494]
      shift-right: [w492] -> w36
      shift-left: w34 -> [w493]
      tunnel: w29 -> [w488]
      tunnel: [w487] -> w26
      stop <- w490 stop-if-true
      # "1."
      # "State Machine"
      n201 = event shown="[3] \"MereniAZpracovaniSwitch\": Value Change" {
        selector: w488 -> [_ _ _ _ _]
        dyn-events: [_ _ _ _ _] -> w487
        timeout: _ -> [_ _ _ _ _]
        tunnel: w494 -> [w501 w505 w517 w522 w526]
        tunnel: w493 -> [w498 w507 w516 w520 w524]
        tunnel: [w495 w508 w511 w519 w523] -> w492
        tunnel: [w502 w506 w513 w521 w525] -> w491
        tunnel: [FALSE TRUE FALSE _ _] -> w490
        event "Cluster 2.Stop Button": Value Change {
          n202 = event-data() -> ()  [unwired: 1 in, 5 out]
          n203 = Enqueue Element(queue=w501, element=Status."Standby" ("Enum"), error in (no error)=w498) -> (queue out=w502:refnum<queue>, error out=w496:errorcluster)  [unwired: 1 in, 1 out]
          n204 = property on="Sync Stop" class="Bool (strict)"(error in=w496, "Val(Sgnl)"=TRUE) -> (error out=w495:errorcluster)  [unwired: 1 in, 1 out]
        }
        event "Exit Button": Value Change {
          n205 = event-data() -> ()  [unwired: 1 in, 5 out]
          n206 = Enqueue Element(queue=w505, element=Status."Exit" ("Enum"), error in (no error)=w507) -> (queue out=w506:refnum<queue>, error out=w508:errorcluster)  [unwired: 1 in, 1 out]
        }
        event "Cluster 2.Record Button": Value Change {
          n207 = event-data() -> ()  [unwired: 1 in, 1 out]
          n208 = Enqueue Element(queue=w517, element=Status."Initialize" ("Enum"), error in (no error)=w516) -> (queue out=w514:refnum<queue>, error out=w512:errorcluster)  [unwired: 1 in, 1 out]
          n209 = Enqueue Element(queue=w514, element=Status."Recording" ("Enum"), error in (no error)=w512) -> (queue out=w513:refnum<queue>, error out=w511:errorcluster)  [unwired: 1 in, 1 out]
        }
        event "MereniAZpracovaniSwitch": Value Change {
          n210 = event-data() -> ()  [unwired: 1 in, 1 out]
          n211 = Enqueue Element(queue=w522, element=Status."Edit", error in (no error)=w520) -> (queue out=w521:refnum<queue>, error out=w519:errorcluster)  [unwired: 1 in, 1 out]
        }
        event User Event {
          n212 = event-data() -> ()  [unwired: 1 in, 1 out]
          n213 = Enqueue Element(queue=w526, element=Status."Standby" ("Enum"), error in (no error)=w524) -> (queue out=w525:refnum<queue>, error out=w523:errorcluster)  [unwired: 1 in, 1 out]
        }
      }
      n214 = Wait Until Next ms Multiple(millisecond multiple=u32 250) -> ()  [unwired: 1 out]
    }
    n215 = Release Queue(queue=w37, error in (no error)=w36) -> (error out=w27:errorcluster)  [unwired: 1 in, 2 out]
    n216 = Unregister For Events(event registration refnum=w26, error in=w27) -> (error out=w25:errorcluster)
    n217 = Destroy User Event(user event=w24, error in=w25) -> ()  [unwired: 1 out]
  }
